vi "제목없음 4.vi"() -> ()   [LabVIEW 2017]
uses:
  <vilib>/Waveform/DWDTOps.llb/DWDT Analog to Digital.vi
  <vilib>/Analysis/NI_AALBase.lvlib
  <vilib>/Waveform/DTblOps.llb/DTbl Digital to Analog.vi
  <vilib>/DAQmx/create/channels.llb/DAQmx Create Channel (DO-Digital Output).vi
  <vilib>/DAQmx/configure/timing.llb/DAQmx Timing (Sample Clock).vi
  <vilib>/DAQmx/write.llb/DAQmx Write (Digital Wfm 1Chan NSamp).vi
panel:
  out "웨이브폼 그래프":waveform(dbl)(graph)
  out "full-scale range (out)":dbl caption="전체 스케일 범위(출력)"
  in  "lines":tag caption="라인"
  in  "device in":tag caption="디바이스 입력"
  out "디지털 웨이브폼 그래프":digitalwaveform(graph)
  in  "sampling rate":dbl=3760000.0 caption="Sampling Frequency" format="%0.2f"
  in  "Pulse length(sec)":dbl=4e-06 format="%#_6p"
  in  "Start Frequency(Hz)":dbl=430000.0 format="%#_6p"
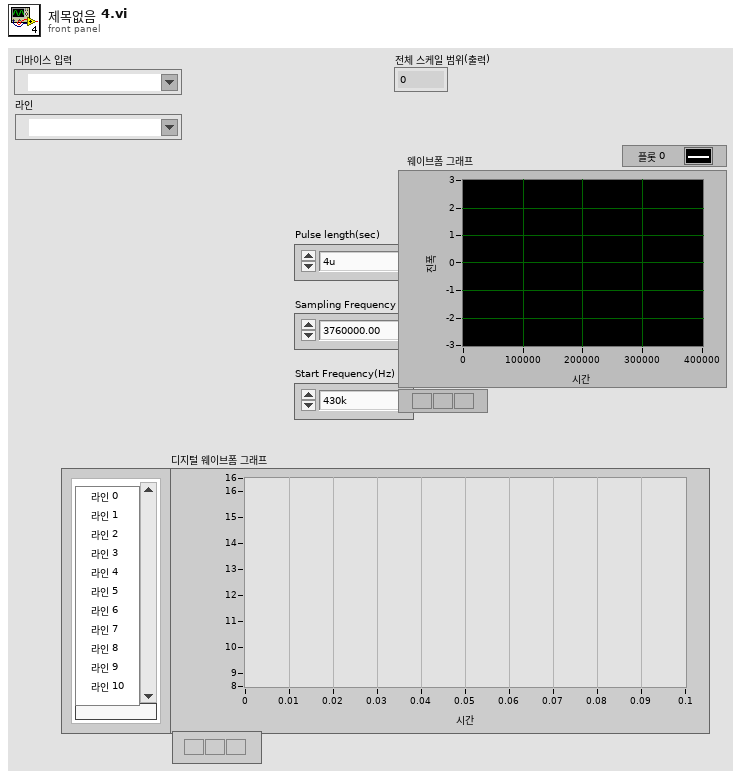
[diagram p1: front panel]
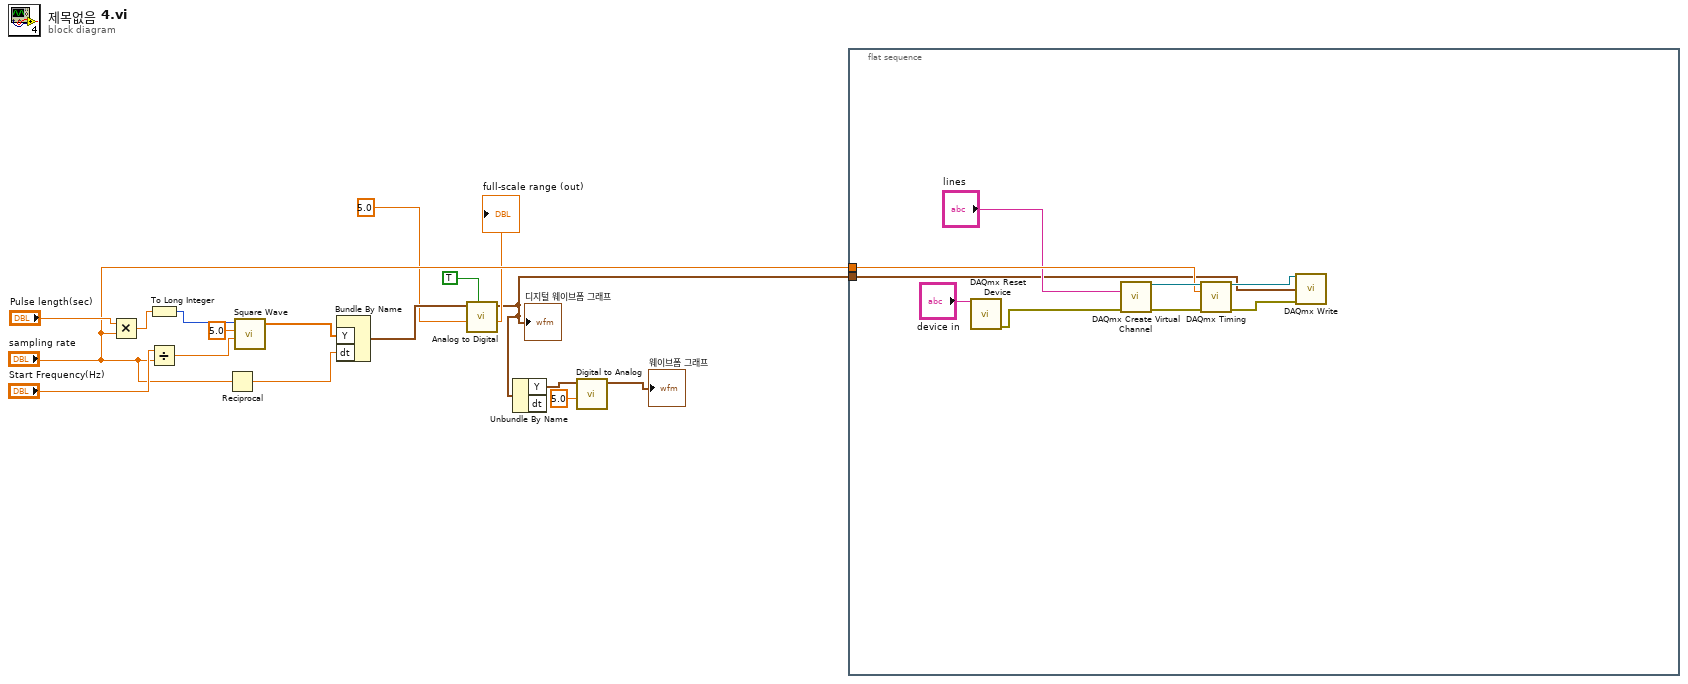
[diagram p0: block diagram]
diagram:
  n1 = Multiply(x="Pulse length(sec)", y="sampling rate") -> (x*y=w14:dbl)
  n2 = To Long Integer(number=w14) -> (32bit integer=w13:i32)
  n3 = Divide(x="Start Frequency(Hz)", y="sampling rate") -> (x/y=w16:dbl)
  n4 = Reciprocal(x="sampling rate") -> (1/x=w11:dbl)
  n5 = call <vilib>:"Square Wave.vi"("samples"=w13, "amplitude"=5.0, "frequency"=w16) -> ("square wave"=w12:dbl[])  [unwired: 3 in, 2 out]
  n6 = Bundle By Name("Y"=w12, "dt"=w11) -> (w10:waveform(dbl))  [unwired: 1 in]
  n7 = call-poly <vilib>:"Analog to Digital.vi"("compress digital (T)"=TRUE, "full-scale range (pk-pk)"=5.0, "analog waveform"=w10) -> ("full-scale range (out)"=→"full-scale range (out)":dbl, "digital waveform"=w4:digitalwaveform)  [unwired: 5 in, 2 out]
  "디지털 웨이브폼 그래프" <- w4
  n8 = Unbundle By Name ("웨이브폼 구성요소 얻기")(w4) -> ("Y"=w1:digitaldata)  [unwired: 1 out]
  n9 = call-poly <vilib>:"Digital to Analog.vi"("full-scale range (pk-pk)"=5.0, "digital table"=w1) -> ("analog waveform"=→"웨이브폼 그래프":waveform(dbl))  [unwired: 6 in, 3 out]
  n10 = flat-sequence {
    tunnel: w4 -> [w18]
    tunnel: "sampling rate" -> [w21]
    frame #0 {
      n11 = call <vilib>:"DAQmx Reset Device.vi"("device in"="device in") -> ("error out"=w20:errorcluster)  [unwired: 1 in, 13 out]
      n12 = call-poly <vilib>:"DAQmx Create Virtual Channel.vi"("lines"="lines", "error in"=w20) -> ("task out"=w25:refnum<k21>, "error out"=w24:errorcluster)  [unwired: 3 in, 9 out]
      n13 = call-poly <vilib>:"DAQmx Timing.vi"("task/channels in"=w25, "rate"=w21, "error in"=w24) -> ("task out"=w22:refnum<k21>, "error out"=w23:errorcluster)  [unwired: 4 in, 7 out]
      n14 = call-poly <vilib>:"DAQmx Write.vi"("task/channels in"=w22, "data"=w18, "error in"=w23) -> ()  [unwired: 10 in, 3 out]
    }
  }
